vi "Perform Action.vi"(8 "error in (no error)":errorcluster, 11 "Scope Simulated in":refnum<class "Scope Simulated.lvclass">) -> (0 "error out":errorcluster, 3 "Scope Simulated out":refnum<class "Scope Simulated.lvclass">)   [LabVIEW 2023]
uses:
  Scope Simulated.lvclass
panel:
  in  "Outtput":variant
  in  "Input":string
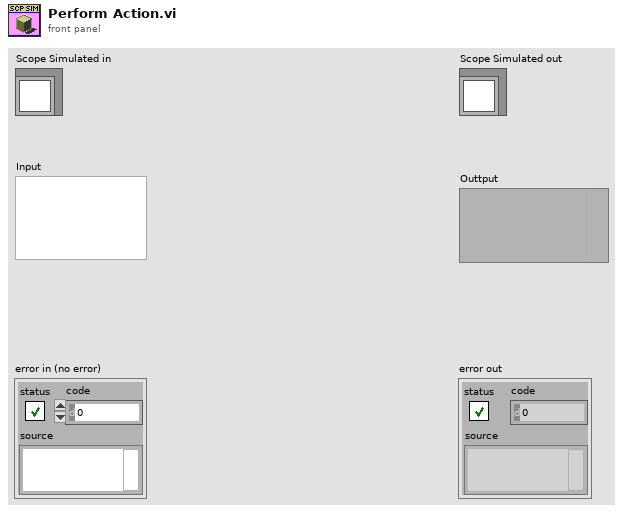
[diagram p1: front panel]
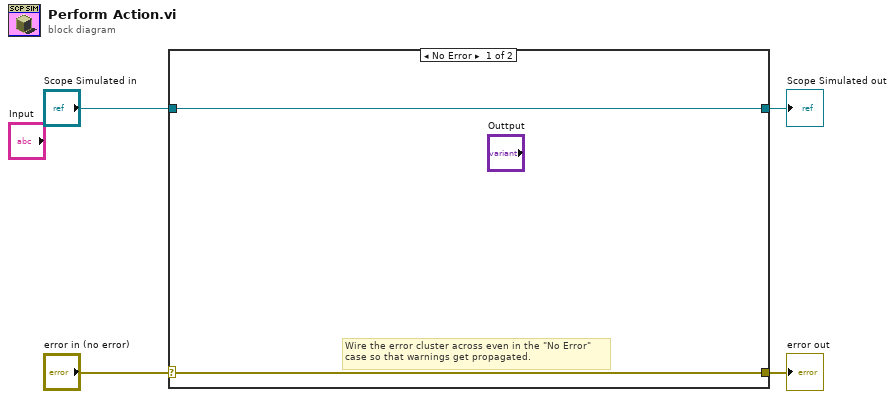
[diagram p0: block diagram]
diagram:
  n1 = case shown="No Error" "error in (no error)" {
    selector: "error in (no error)" -> [w5 w8]
    tunnel: [w5 w8] -> w3
    tunnel: [w6 w7] -> w1
    tunnel: "Scope Simulated in" -> [w6 w7]
    frame No Error {
      # "Wire the error cluster across even in the \"No Error\"\ncase so that warnings get propagated."
    }
    frame Error {
    }
  }
  "error out" <- w3
  "Scope Simulated out" <- w1
